vi "StreapDecode.vi"(4 "EmptyDataIn":i32[](array[numeric]) format="%.0x", 6 "STREAP":i32[](array[numeric]), 7 "VALUE":i32[](array[numeric])) -> (0 "X2":i32[](array[numeric]), 1 "X1":i32[](array[numeric]), 2 "Y2":i32[](array[numeric]), 3 "Y1":i32[](array[numeric]))   [LabVIEW 2014]
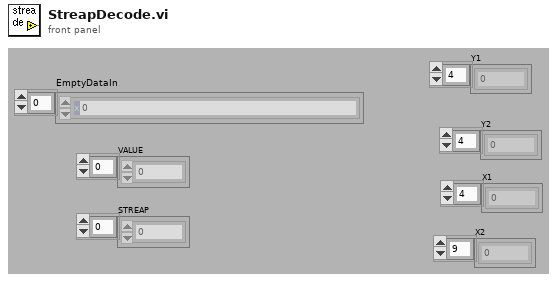
[diagram p1: front panel]
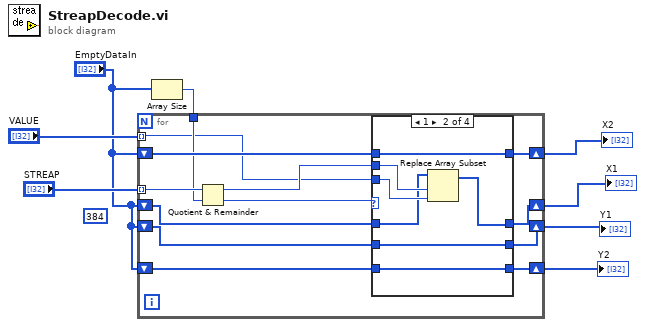
[diagram p0: block diagram]
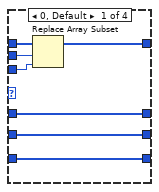
[diagram p2: hidden frame]
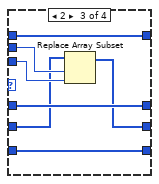
[diagram p3: hidden frame]
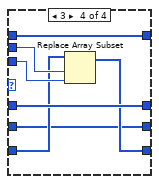
[diagram p4: hidden frame]
diagram:
  (unwired) 384
  n1 = Array Size(array="EmptyDataIn") -> (size(s)=w3:i32)
  n2 = for {
    tunnel: "VALUE" -> [w9] mode=indexing
    tunnel: "STREAP" -> [w21] mode=indexing
    tunnel: w3 -> [w10]
    shift-right: [w14] -> w6
    shift-left: "EmptyDataIn" -> [w20]
    shift-right: [w13] -> w1
    shift-left: "EmptyDataIn" -> [w17]
    shift-right: [w12] -> w2
    shift-left: "EmptyDataIn" -> [w16]
    shift-right: [w11] -> w5
    shift-left: "EmptyDataIn" -> [w15]
    n3 = Quotient & Remainder(x=w21, y=w10) -> (x-y*floor(x/y)=w19:i32, floor(x/y)=w18:i32)
    n4 = case shown="1" w18 {
      tunnel: w20 -> [w28 w29 w39 w47]
      tunnel: w19 -> [w27 w35 w42 w49]
      tunnel: w9 -> [w26 w34 w41 w48]
      tunnel: w17 -> [w25 w31 w38 w46]
      tunnel: [w25 w30 w38 w46] -> w13
      tunnel: w16 -> [w24 w33 w37 w43]
      tunnel: [w24 w33 w36 w43] -> w12
      tunnel: w15 -> [w23 w32 w40 w45]
      tunnel: [w23 w32 w40 w44] -> w11
      tunnel: [w22 w29 w39 w47] -> w14
      frame 0, Default {
        n5 = Replace Array Subset(array=w28, new element=w26, index=w27) -> (w22:i32[])
      }
      frame 1 {
        n6 = Replace Array Subset(array=w31, new element=w34, index=w35) -> (w30:i32[])
      }
      frame 2 {
        n7 = Replace Array Subset(array=w37, new element=w41, index=w42) -> (w36:i32[])
      }
      frame 3 {
        n8 = Replace Array Subset(array=w45, new element=w48, index=w49) -> (w44:i32[])
      }
    }
  }
  "X2" <- w6
  "X1" <- w1
  "Y1" <- w2
  "Y2" <- w5
